vi "Change Windows Title.vi"(8 "error in (no error)":errorcluster, 10 "Front Panel Window:Title":string, 11 "UnitTestEngine in":refnum<class "UnitTestEngine.lvclass">) -> (0 "error out":errorcluster, 3 "UnitTestEngine out":refnum<class "UnitTestEngine.lvclass">)   [LabVIEW 2019, in "UnitTestEngine.lvlib" / "UnitTestEngine.lvclass"]
uses:
  UnitTestEngine.lvclass
  UnitTestEngine.lvclass/UnitTestEngine.ctl
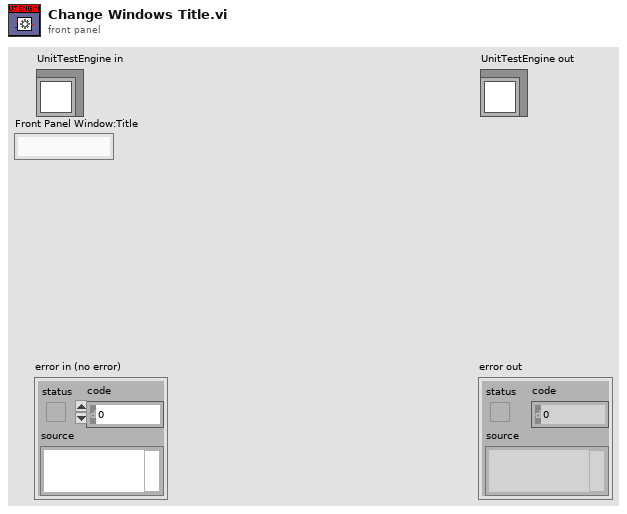
[diagram p1: front panel]
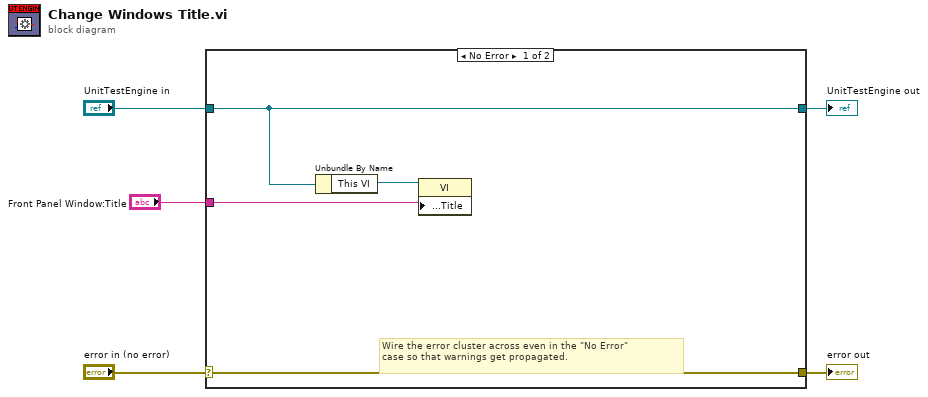
[diagram p0: block diagram]
diagram:
  n1 = case shown="No Error" "error in (no error)" {
    selector: "error in (no error)" -> [w9 w11]
    tunnel: [w9 w11] -> w4
    tunnel: [w8 w10] -> w2
    tunnel: "UnitTestEngine in" -> [w8 w10]
    tunnel: "Front Panel Window:Title" -> [w6 _]
    frame No Error {
      # "Wire the error cluster across even in the \"No Error\"\ncase so that warnings get propagated."
      n2 = Unbundle By Name(w8) -> ("This VI"=w7:refnum<vi>)
      n3 = property class="VI"(reference=w7, "Front Panel.Title"=w6) -> ()  [unwired: 1 in, 2 out]
    }
    frame Error {
    }
  }
  "error out" <- w4
  "UnitTestEngine out" <- w2
